vi "Destroy.vi"(0 "ClassWriterNative":refnum<class "ClassWriterNative.lvclass">, 5 "error in (no error)":errorcluster) -> (19 "error out":errorcluster)   [LabVIEW 2020, in "ClassWriterNative.lvclass"]
doc: "Destroys a ClassWriterNative object created with a ClassWriterNative constructor VI.\n\n[GOOP 2.0.16]"
uses:
  ClassWriterNative.lvclass
  ClassWriterNative.lvclass/ClassWriterNative.ctl
  Provider_BaseClassInterface/ClassWriter_class/ClassWriter.lvclass
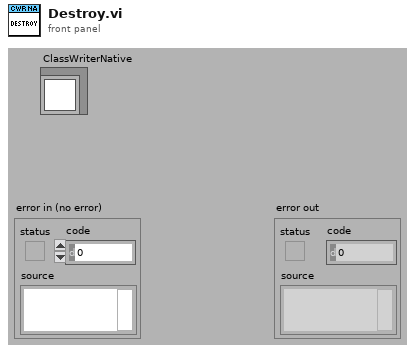
[diagram p1: front panel]
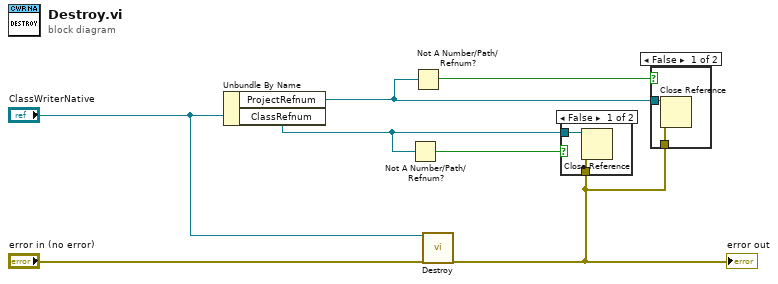
[diagram p0: block diagram]
diagram:
  n1 = Unbundle By Name("ClassWriterNative") -> ("ProjectRefnum"=w4:refnum<vi>, "ClassRefnum"=w3:refnum<vi>)
  n2 = Not A Number/Path/Refnum?(number/path/refnum=w3) -> (NaN/Path/Refnum?=w1:bool)
  n3 = Not A Number/Path/Refnum?(number/path/refnum=w4) -> (NaN/Path/Refnum?=w2:bool)
  n4 = call-parent "Destroy.vi"("ClassWriter.lvclass"="ClassWriterNative", "error in (no error)"="error in (no error)") -> ("error out"=w5:errorcluster)  [unwired: 17 in]
  "error out" <- w5
  n5 = case shown="False" w1 {
    tunnel: w5 -> [w9 _]
    tunnel: w3 -> [w8 _]
    frame False {
      n6 = Close Reference(reference=w8, error in (no error)=w9) -> ()  [unwired: 1 out]
    }
    frame True {
    }
  }
  n7 = case shown="False" w2 {
    tunnel: w5 -> [w11 _]
    tunnel: w4 -> [w10 _]
    frame False {
      n8 = Close Reference(reference=w10, error in (no error)=w11) -> ()  [unwired: 1 out]
    }
    frame True {
    }
  }
